vi "lijnvolgen_deel2 (SubVI).vi"(9 "rechtermotor":dbl, 10 "linkermotor":dbl, 11 "array":dbl[](array[numeric])) -> (1 "rechtermotor na":dbl, 2 "linkermotor na":dbl)   [LabVIEW 2019]
uses:
  <vilib>/addons/control/pid/NI_PID_pid.lvlib
  <vilib>/addons/control/pid/pid.llb/PID (DBL).vi
  <vilib>/myRIO/Instrument Drivers/Onboard IO/PWM/typedefs/PWM Configuration.ctl
  <vilib>/myRIO/Instrument Drivers/Onboard IO/PWM/PWM.lvlib
  <vilib>/myRIO/Common/Instrument Driver Framework/myRIO v1.0/PWM/typedefs/PWM Channels Enum.ctl
  <vilib>/myRIO/Common/Instrument Driver Framework/Utilities/typedefs/Generic FPGA Reference.ctl
  <vilib>/myRIO/Common/Instrument Driver Framework/Utilities/typedefs/myRIO v1.0 Reference.ctl
  <vilib>/myRIO/Common/Instrument Driver Framework/Utilities/typedefs/Hardware Version Enum.ctl
  <vilib>/myRIO/Common/Instrument Driver Framework/Utilities/typedefs/myRIO Generic Hardware Reference.ctl
  <vilib>/myRIO/Instrument Drivers/Onboard IO/PWM/typedefs/PWM Reference.ctl
  <vilib>/myRIO/Instrument Drivers/Onboard IO/PWM/vis/Set Duty Cycle and Frequency.vi
  <vilib>/userDefined/High Color/nirio_resource_hc.ctl
  <vilib>/myRIO/Common/Instrument Driver Framework/myRIO v1.0/PWM/vis/myRIO v1.1 Open PWM.vi
  <vilib>/myRIO/Instrument Drivers/Onboard IO/PWM/vis/myRIO PWM Open.xnode
  <vilib>/myRIO/Common/Instrument Driver Framework/Utilities/vis/Is FPGA Ref Available.vi
  <vilib>/myRIO/Express VI/Onboard IO/PWM/PWM Express VI.xnode
panel:
  out "output":dbl format="%.2f"
  out "Gauge 2":cluster{dbl, dbl}(knob)={0.0, 8.725388533162729} scale=-0.5..0.5
  in  "output range":cluster{"output high":dbl, "output low":dbl}={"output high"=100.0, "output low"=-100.0} {"output low" format="%.2f"; "output high" format="%.2f"}
  in  "PID gains":T1={"proportional gain (Kc)"=1.0, "integral time (Ti, min)"=0.01, "derivative time (Td, min)"=0.0} {"derivative time (Td, min)" format="%.3f"; "integral time (Ti, min)" format="%.3f"; "proportional gain (Kc)" format="%.3f"}
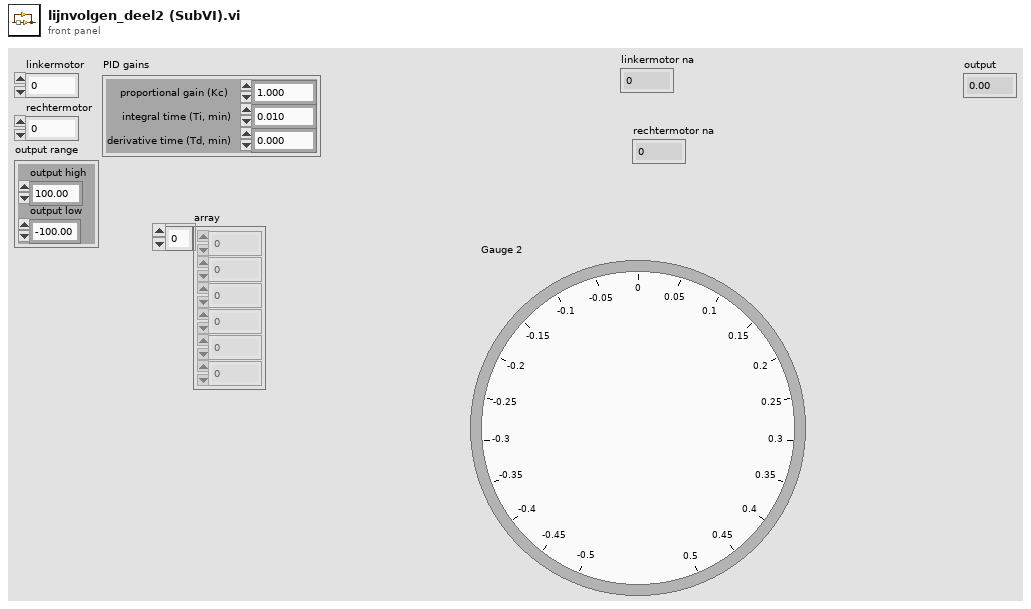
[diagram p1: front panel]
types:
  T1 = cluster{"proportional gain (Kc)":dbl, "integral time (Ti, min)":dbl, "derivative time (Td, min)":dbl}
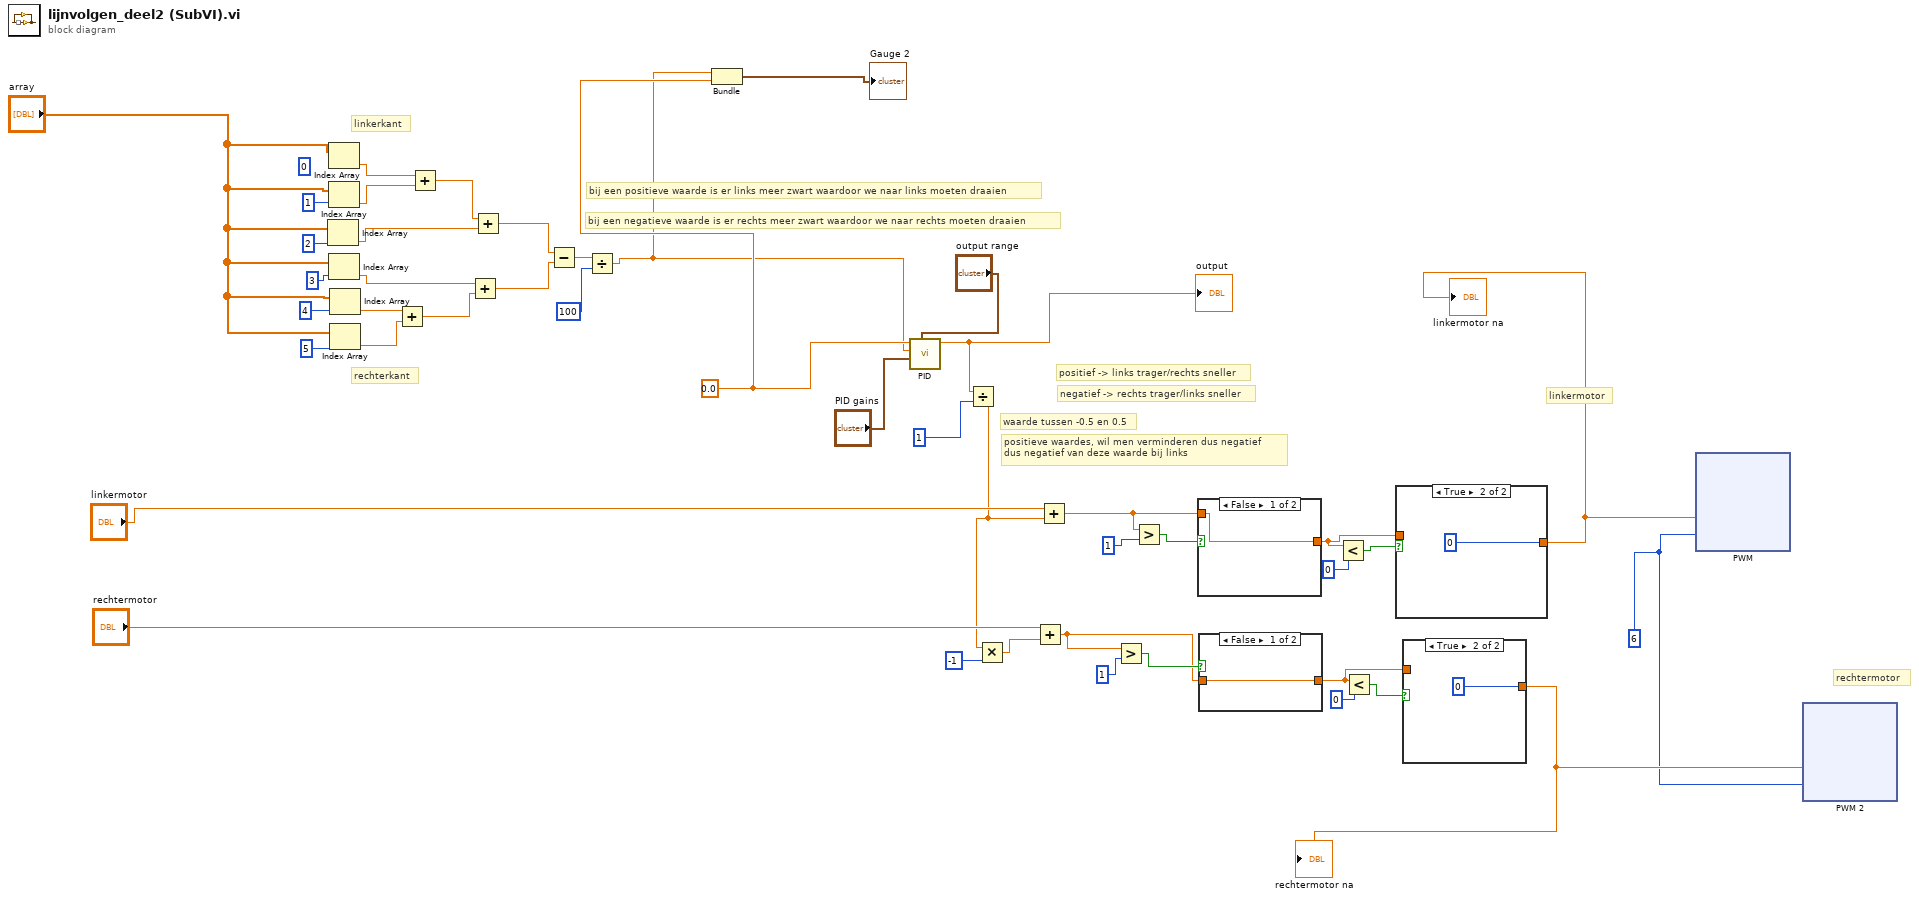
[diagram p0: block diagram]
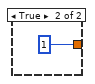
[diagram p4: hidden frame]
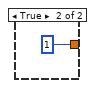
[diagram p5: hidden frame]
diagram:
  w1 = 6
  (unwired) 0
  w26 = 0.0 ("setpoint")
  # "rechtermotor"
  # "linkermotor"
  # "positieve waardes, wil men verminderen dus negatief \ndus negatief van deze waarde bij links"
  # "waarde tussen -0.5 en 0.5"
  # "negatief -> rechts trager/links sneller"
  # "positief -> links trager/rechts sneller"
  # "bij een negatieve waarde is er rechts meer zwart waardoor we naar rechts moeten draaien"
  # "bij een positieve waarde is er links meer zwart waardoor we naar links moeten draaien"
  # "rechterkant"
  # "linkerkant"
  n1 = Index Array(array="array", index=2) -> (element=w38:dbl)
  n2 = Index Array(array="array") -> (element=w40:dbl)  [unwired: 1 in]
  n3 = Index Array(array="array", index=1) -> (element=w39:dbl)
  n4 = Index Array(array="array", index=3) -> (element=w33:dbl)
  n5 = Index Array(array="array", index=4) -> (element=w36:dbl)
  n6 = Index Array(array="array", index=5) -> (element=w35:dbl)
  n7 = Add(x=w36, y=w35) -> (x+y=w34:dbl)
  n8 = Add(x=w40, y=w39) -> (x+y=w37:dbl)
  n9 = Add(x=w33, y=w34) -> (x+y=w31:dbl)
  n10 = Add(x=w37, y=w38) -> (x+y=w32:dbl)
  n11 = Subtract(x=w32, y=w31) -> (x-y=w17:dbl)
  n12 = Divide(x=w17, y=100) -> (x/y=w18:dbl)
  n13 = Bundle(w18, "setpoint"=w26) -> (→"Gauge 2":cluster{dbl, "setpoint":dbl})  [unwired: 1 in]
  n14 = call-poly <vilib>:"PID.vi"("output range"="output range", "PID gains"="PID gains", "process variable"=w18, "setpoint"=w26) -> ("output"=w19:dbl)  [unwired: 6 in, 1 out]
  "output" <- w19
  n15 = Divide(x=w19, y=1) -> (x/y=w21:dbl)
  n16 = Multiply(x=w21, y=-1) -> (x*y=w22:dbl)
  n17 = Add(x="rechtermotor", y=w22) -> (x+y=w11:dbl)
  n18 = Add(x="linkermotor", y=w21) -> (x+y=w10:dbl)
  n19 = Greater?(x=w11, y=1) -> (0:w13:bool)
  n20 = Greater?(x=w10, y=1) -> (0:w14:bool)
  n21 = case shown="False" w14 {
    tunnel: [w46 1] -> w6
    tunnel: w10 -> [w46 _]
    frame False {
    }
    frame True {
    }
  }
  n22 = case shown="False" w13 {
    tunnel: [w48 1] -> w2
    tunnel: w11 -> [w48 _]
    frame False {
    }
    frame True {
    }
  }
  n23 = Less?(x=w6, y=0) -> (x < y?=w9:bool)
  n24 = Less?(x=w2, y=0) -> (x < y?=w4:bool)
  n25 = case shown="True" w9 {
    tunnel: [w50 0] -> w7
    tunnel: w6 -> [w50 _]
    frame False {
    }
    frame True {
    }
  }
  "linkermotor na" <- w7
  n26 = case shown="True" w4 {
    tunnel: [w52 0] -> w3
    tunnel: w2 -> [w52 _]
    frame False {
    }
    frame True {
    }
  }
  "rechtermotor na" <- w3
  n27 = xnode "PWM"("Duty Cycle"=w7, "Frequency [Hz]"=w1) -> ()  [unwired: 1 in, 1 out]
  n28 = xnode "PWM 2"("Duty Cycle"=w3, "Frequency [Hz]"=w1) -> ()  [unwired: 1 in, 1 out]
